vi "ProcessDataV1729A.vi"(7 "Module":string, 9 "Buffer":u32[](array[numeric]), 10 "TRIG_REC":u32, 11 "# Samples after Trig":u16) -> (0 "Channel Data":sgl[][](array[numeric]), 3 "Vernier Data":u16[](array[numeric]))   [LabVIEW 2014]
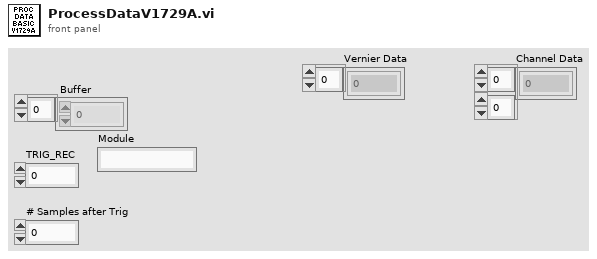
[diagram p1: front panel]
types:
  T1 = cluster{"MAXVER_0":u16, "MINVER_0":u16, "MAXVER_1":u16, "MINVER_1":u16, "MAXVER_2":u16, "MINVER_2":u16, "MAXVER_3":u16, "MINVER_3":u16}
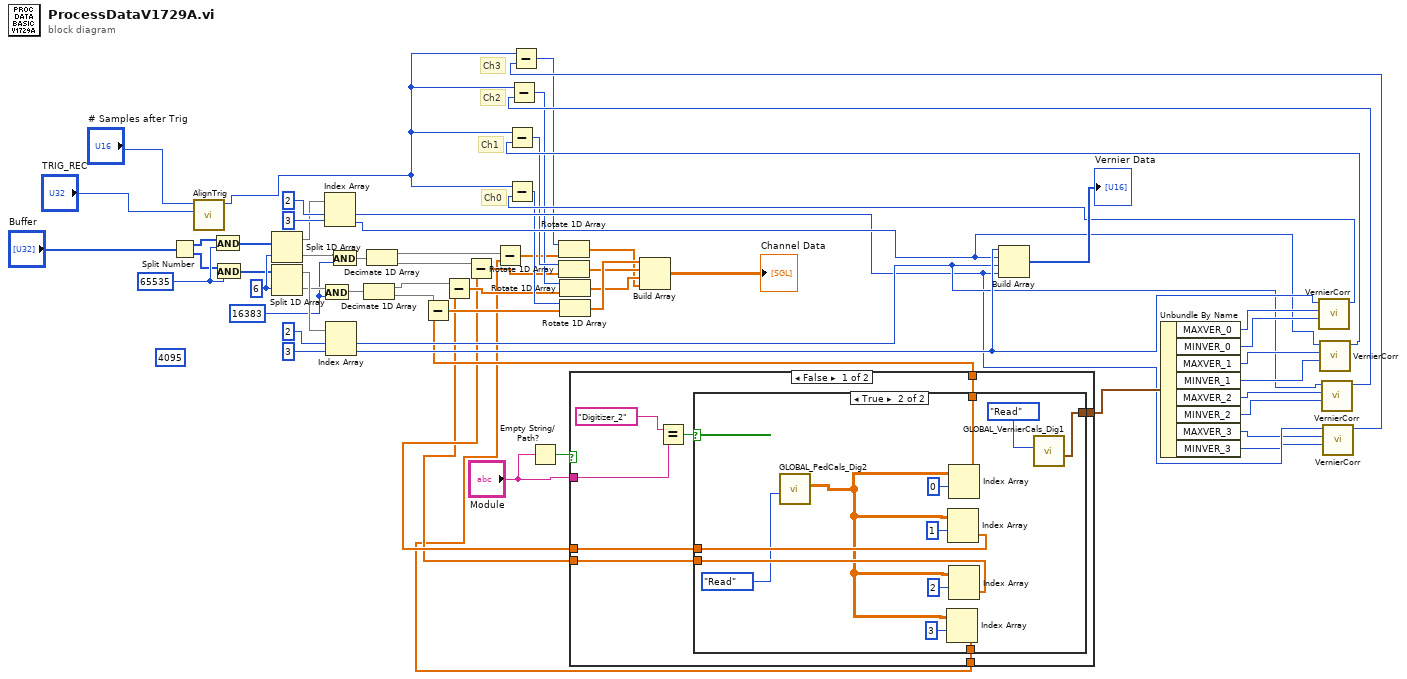
[diagram p0: block diagram]
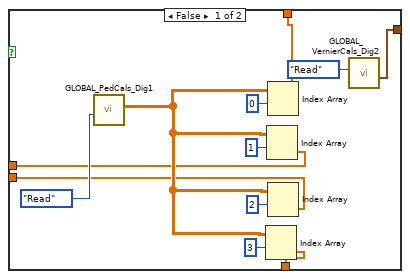
[diagram p2: hidden frame]
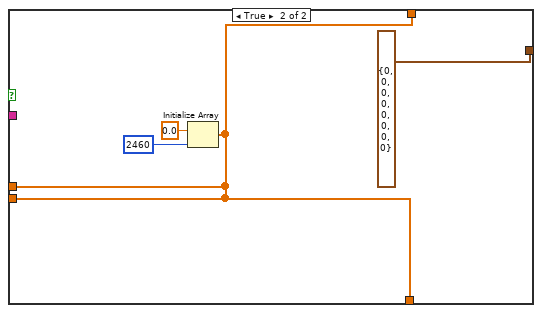
[diagram p3: hidden frame]
diagram:
  w37 = u16 16383 ("Numeric")
  (unwired) u16 4095 ("Numeric")
  w56 = 6 ("index")
  w53 = u16 65535 ("Numeric")
  # "Ch3"
  # "Ch2"
  # "Ch1"
  # "Ch0"
  n1 = Split Number(x="Buffer") -> (hi(x)=w52:u16[], lo(x)=w51:u16[])
  n2 = call "AlignTrig.vi"("TRIG_REC"="TRIG_REC", "# Samples after Trig"="# Samples after Trig") -> ("Offset"=w18:i16)  [unwired: 9 in]
  n3 = And(x=w52, y=w53) -> (x .and. y?=w54:u16[])
  n4 = And(x=w51, y=w53) -> (x .and. y?=w55:u16[])
  n5 = Split 1D Array(array=w54, index=w56) -> (first subarray=w57:u16[], second subarray=w39:u16[])
  n6 = Split 1D Array(array=w55, index=w56) -> (first subarray=w60:u16[], second subarray=w40:u16[])
  n7 = And(x=w40, y=w37) -> (x .and. y?=w41:u16[])
  n8 = Index Array(array=w57, index #1=2 ("index"), index #2=3 ("index")) -> (element #1=w24:u16, element #2=w30:u16)
  n9 = Index Array(array=w60, index #1=2 ("index"), index #2=3 ("index")) -> (element #1=w27:u16, element #2=w33:u16)
  n10 = And(x=w39, y=w37) -> (x .and. y?=w38:u16[])
  n11 = Decimate 1D Array(w41) -> (w10:u16[], w12:u16[])
  n12 = Decimate 1D Array(w38) -> (w6:u16[], w8:u16[])
  n13 = Empty String/Path?(string/path="Module") -> (empty?=w35:bool)
  n14 = case shown="False" w35 {
    tunnel: "Module" -> [w69 _]
    tunnel: [w67 T1 {"MAXVER_0"=0, "MINVER_0"=0, "MAXVER_1"=0, "MINVER_1"=0, "MAXVER_2"=0, "MINVER_2"=0, "MAXVER_3"=0, "MINVER_3"=0} ("Digitizer1 OUT")] -> w34
    tunnel: [w66 w95] -> w4
    tunnel: [w65 w95] -> w3
    tunnel: [w64 w95] -> w2
    tunnel: [w63 w95] -> w1
    frame False {
      n15 = Equal?(x="Digitizer_2" ("Module"), y=w69) -> (x = y?=w68:bool)
      n16 = case shown="True" w68 {
        tunnel: [w82 w93] -> w67
        tunnel: [w74 w88] -> w66
        tunnel: [w73 w87] -> w65
        tunnel: [w72 w86] -> w64
        tunnel: [w71 w85] -> w63
        frame False {
          n17 = call "GLOBAL_PedCals_Dig1.vi"("State"=enum16{"Initialise", "Write", "Read"}."Read") -> ("Data Out"=w80:dbl[][])  [unwired: 10 in]
          n18 = Index Array(array=w80, index (row)=3) -> (element=w71:dbl[])  [unwired: 1 in]
          n19 = Index Array(array=w80, index (row)=1) -> (element=w73:dbl[])  [unwired: 1 in]
          n20 = Index Array(array=w80, index (row)=0) -> (element=w74:dbl[])  [unwired: 1 in]
          n21 = Index Array(array=w80, index (row)=2) -> (element=w72:dbl[])  [unwired: 1 in]
          n22 = call "GLOBAL_VernierCals_Dig2.vi"("State"=enum16{"Initialise", "Write", "Read"}."Read") -> ("Digitizer2 OUT"=w82:T1)  [unwired: 10 in]
        }
        frame True {
          n23 = call "GLOBAL_PedCals_Dig2.vi"("State"=enum16{"Initialise", "Write", "Read"}."Read") -> ("Data Out"=w84:dbl[][])  [unwired: 10 in]
          n24 = Index Array(array=w84, index (row)=3) -> (element=w85:dbl[])  [unwired: 1 in]
          n25 = Index Array(array=w84, index (row)=1) -> (element=w87:dbl[])  [unwired: 1 in]
          n26 = Index Array(array=w84, index (row)=0) -> (element=w88:dbl[])  [unwired: 1 in]
          n27 = Index Array(array=w84, index (row)=2) -> (element=w86:dbl[])  [unwired: 1 in]
          n28 = call "GLOBAL_VernierCals_Dig1.vi"("State"=enum16{"Initialise", "Write", "Read"}."Read") -> ("Digitizer1 OUT"=w93:T1)  [unwired: 10 in]
        }
      }
    }
    frame True {
      n29 = Initialize Array(0.0 ("element"), 2460 ("dimension size")) -> (w95:dbl[])
    }
  }
  n30 = Subtract(x=w12, y=w4) -> (x-y=w11:dbl[])
  n31 = Subtract(x=w10, y=w2) -> (x-y=w9:dbl[])
  n32 = Subtract(x=w8, y=w3) -> (x-y=w7:dbl[])
  n33 = Subtract(x=w6, y=w1) -> (x-y=w5:dbl[])
  n34 = Build Array(w33, w30, w27, w24) -> (→"Vernier Data":u16[])
  n35 = Unbundle By Name(w34) -> ("MAXVER_0"=w32:u16, "MINVER_0"=w31:u16, "MAXVER_1"=w29:u16, "MINVER_1"=w28:u16, "MAXVER_2"=w26:u16, "MINVER_2"=w25:u16, "MAXVER_3"=w23:u16, "MINVER_3"=w22:u16)
  n36 = call "VernierCorr.vi"("MINVER"=w31, "MAXVER"=w32, "Numeric"=w33) -> ("VernierCorr"=w21:u16)  [unwired: 8 in]
  n37 = Subtract(x=w18, y=w21) -> (x-y=w14:u16)
  n38 = Rotate 1D Array(1:w11, 2:w14) -> (0:w47:dbl[])
  n39 = call "VernierCorr.vi"("MINVER"=w28, "MAXVER"=w29, "Numeric"=w30) -> ("VernierCorr"=w20:u16)  [unwired: 8 in]
  n40 = Subtract(x=w18, y=w20) -> (x-y=w16:u16)
  n41 = Rotate 1D Array(1:w7, 2:w16) -> (0:w46:dbl[])
  n42 = call "VernierCorr.vi"("MINVER"=w25, "MAXVER"=w26, "Numeric"=w27) -> ("VernierCorr"=w19:u16)  [unwired: 8 in]
  n43 = Subtract(x=w18, y=w19) -> (x-y=w15:u16)
  n44 = Rotate 1D Array(1:w9, 2:w15) -> (0:w45:dbl[])
  n45 = call "VernierCorr.vi"("MINVER"=w22, "MAXVER"=w23, "Numeric"=w24) -> ("VernierCorr"=w17:u16)  [unwired: 8 in]
  n46 = Subtract(x=w18, y=w17) -> (x-y=w13:u16)
  n47 = Rotate 1D Array(1:w5, 2:w13) -> (0:w44:dbl[])
  n48 = Build Array(w47, w46, w45, w44) -> (→"Channel Data":dbl[][])
